vi "Rings with Colors.vi"(0 "Number of Rings":i32=4, 5 "Separation (angle)":dbl=5.0, 7 "Colour Option":T1(ring), 11 "error in (no error)":errorcluster) -> (15 "error out":errorcluster)   [LabVIEW 2017]
doc: "To draw rings on the spherical object."
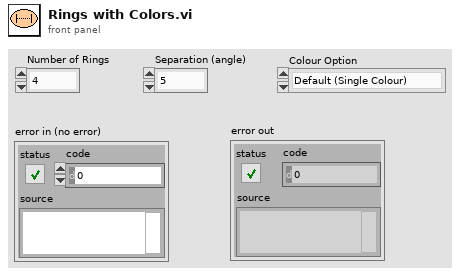
[diagram p1: front panel]
types:
  T1 = enum16{"Default (Single Colour)", "Rings with Colours"}
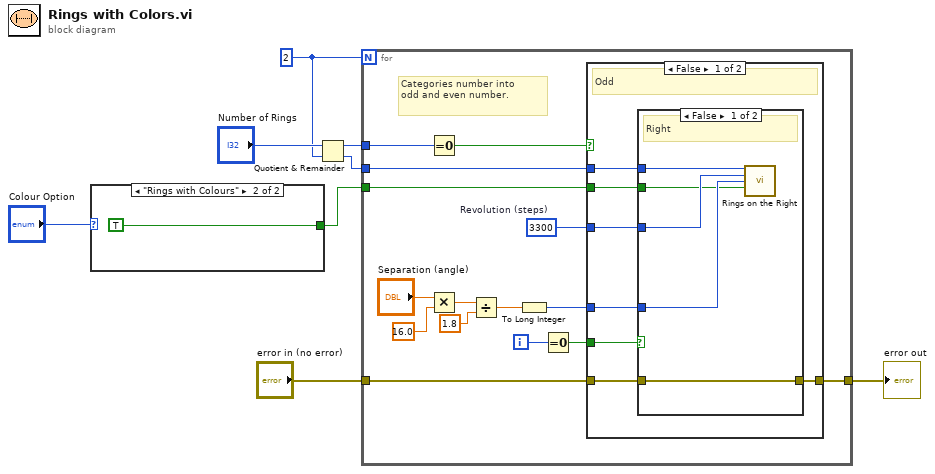
[diagram p0: block diagram]
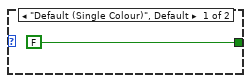
[diagram p2: hidden frame]
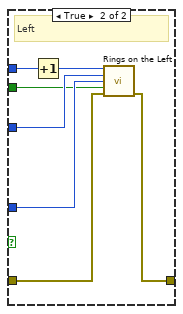
[diagram p3: hidden frame]
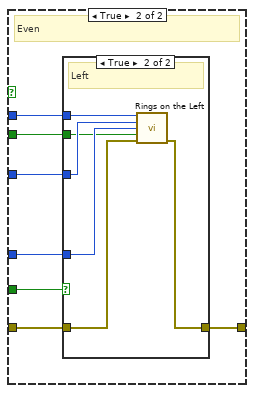
[diagram p4: hidden frame]
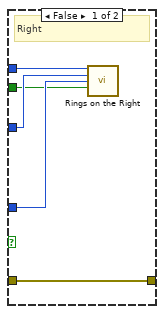
[diagram p5: hidden frame]
diagram:
  w1 = 2 ("y")
  n1 = case shown="\"Rings with Colours\"" "Colour Option" {
    tunnel: [FALSE TRUE] -> w5
    frame "Default (Single Colour)", Default {
    }
    frame "Rings with Colours" {
    }
  }
  n2 = Quotient & Remainder(x="Number of Rings", y=w1) -> (x-y*floor(x/y)=w7:i32, floor(x/y)=w6:i32)
  n3 = for {
    N: w1 -> [_]
    tunnel: w6 -> [w23]
    tunnel: w7 -> [w22]
    tunnel: w5 -> [w13]
    tunnel: "error in (no error)" -> [w12]
    tunnel: [w11] -> w2
    i -> [w25]
    w20 = 3300  # Revolution (steps)
    # "Categories number into\nodd and even number."
    n4 = Equal To 0?(x=w22) -> (x = 0?=w21:bool)
    n5 = Multiply(x="Separation (angle)", y=16.0) -> (x*y=w17:dbl)
    n6 = Divide(x=w17, y=1.8) -> (x/y=w15:dbl)
    n7 = To Long Integer(number=w15) -> (32bit integer=w14:i32)
    n8 = Equal To 0?(x=w25) -> (x = 0?=w24:bool)
    n9 = case shown="False" w21 {
      tunnel: w24 -> [w29 w51]
      tunnel: w23 -> [w32 w48]
      tunnel: w14 -> [w30 w50]
      tunnel: w20 -> [w31 w49]
      tunnel: w13 -> [w28 w47]
      tunnel: w12 -> [w27 w46]
      tunnel: [w26 w45] -> w11
      frame False {
        # "Odd"
        n10 = case shown="False" w29 {
          tunnel: w32 -> [w37 w44]
          tunnel: w31 -> [w36 w43]
          tunnel: w30 -> [w35 w42]
          tunnel: w28 -> [w34 w40]
          tunnel: [w33 w38] -> w26
          tunnel: w27 -> [w33 w39]
          frame False {
            # "Right"
            n11 = call "Rings on the Right.vi"("Iteration"=w37, "Revolution (steps)"=w36, "Separation (angle)"=w35, "Change colours?"=w34) -> ()  [unwired: 11 in, 1 out]
          }
          frame True {
            # "Left"
            n12 = Increment(x=w44) -> (x+1=w41:i32)
            n13 = call "Rings on the Left.vi"("Iteration"=w41, "Revolution (steps)"=w43, "Separation (angle)"=w42, "Change colours?"=w40, "error in (no error)"=w39) -> ("error out"=w38:errorcluster)  [unwired: 10 in]
          }
        }
      }
      frame True {
        # "Even"
        n14 = case shown="True" w51 {
          tunnel: w48 -> [w56 w62]
          tunnel: w49 -> [w55 w61]
          tunnel: w50 -> [w54 w60]
          tunnel: w47 -> [w53 w59]
          tunnel: [w52 w57] -> w45
          tunnel: w46 -> [w52 w58]
          frame False {
            # "Right"
            n15 = call "Rings on the Right.vi"("Iteration"=w56, "Revolution (steps)"=w55, "Separation (angle)"=w54, "Change colours?"=w53) -> ()  [unwired: 11 in, 1 out]
          }
          frame True {
            # "Left"
            n16 = call "Rings on the Left.vi"("Iteration"=w62, "Revolution (steps)"=w61, "Separation (angle)"=w60, "Change colours?"=w59, "error in (no error)"=w58) -> ("error out"=w57:errorcluster)  [unwired: 10 in]
          }
        }
      }
    }
  }
  "error out" <- w2
